vi "Convert ITX Experiment Folder.vi"(8 "error in (no error)":errorcluster, 11 "Folder Path":path) -> (0 "error out":errorcluster)   [LabVIEW 2016, in "Conversion.lvclass"]
uses:
  Conversion.lvclass
  Conversion.lvclass/Conversion.ctl
  Data/Data.lvclass
panel:
  in  "OK":bool
  in  "Additional Notes?":string
  out "Elapsed Time (s)":dbl
  out "Numeric":i32
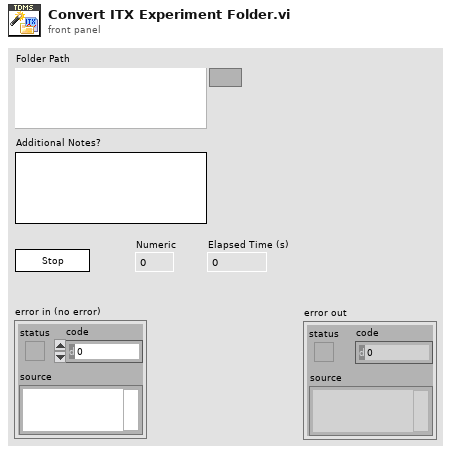
[diagram p1: front panel]
types:
  T1 = enum32{"Invalid", "Standard", "Closed", "Hidden", "Minimized", "Maximized"}
  T2 = enum32{"invalid app kind", "Development System", "Run Time System", "Student Edition", "Embedded LabVIEW", "Evaluation", "Custom"}
  T3 = cluster{"Core":cluster{"Current VI Reference":refnum<vi>, "Close Panel on Exit?":bool}, "Conversion.lvclass":refnum<class "Conversion.lvclass">, "Start Time":dbl, "End Time":dbl, "File Index":i32, "Number of Files":i32, "Log File Path":path}
  T4 = cluster{"Current VI Reference":refnum<vi>, "Close Panel on Exit?":bool}
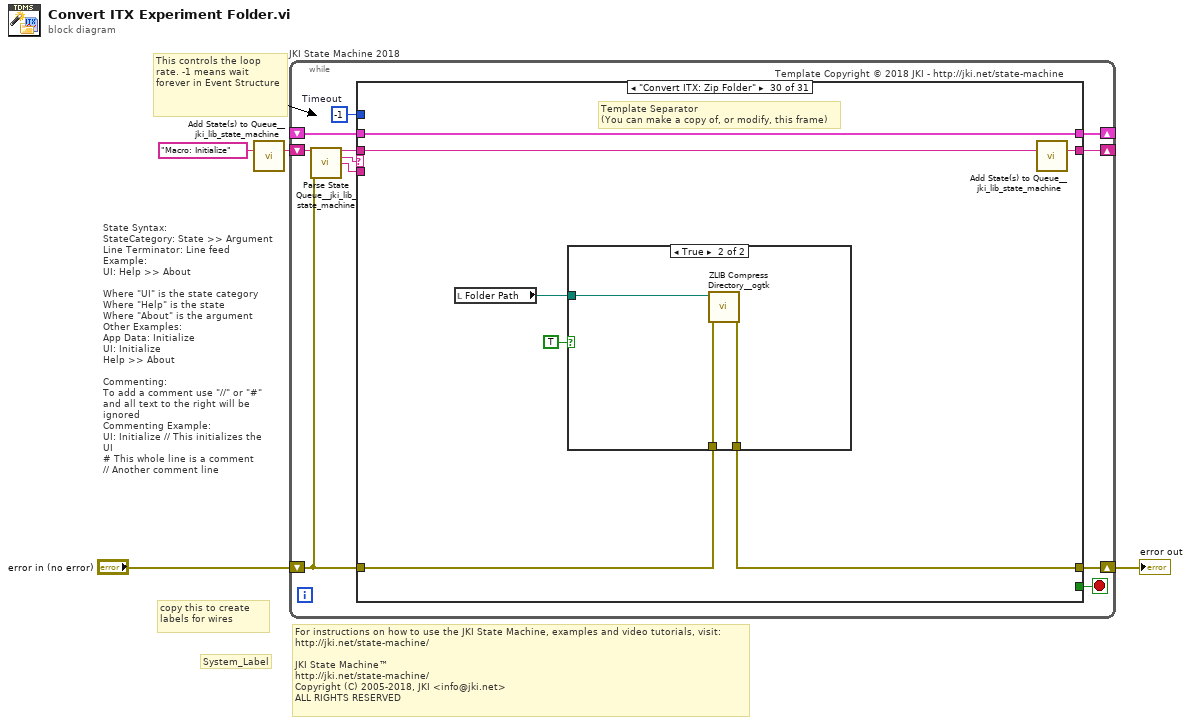
[diagram p0: block diagram]
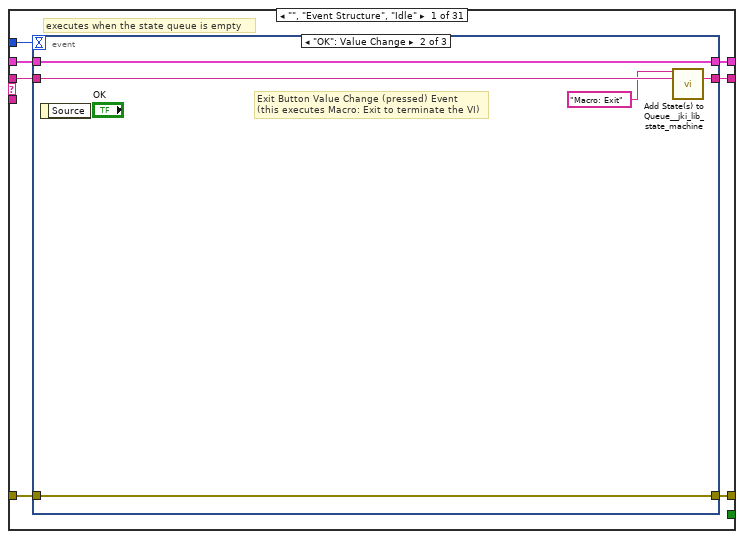
[diagram p2: hidden frame]
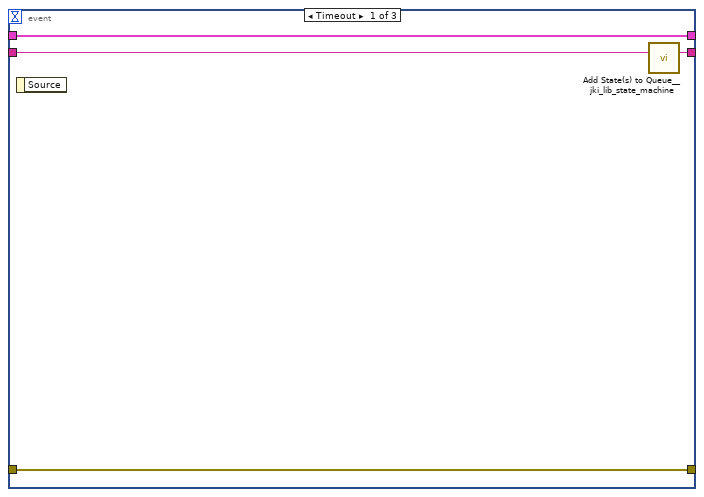
[diagram p3: hidden frame]
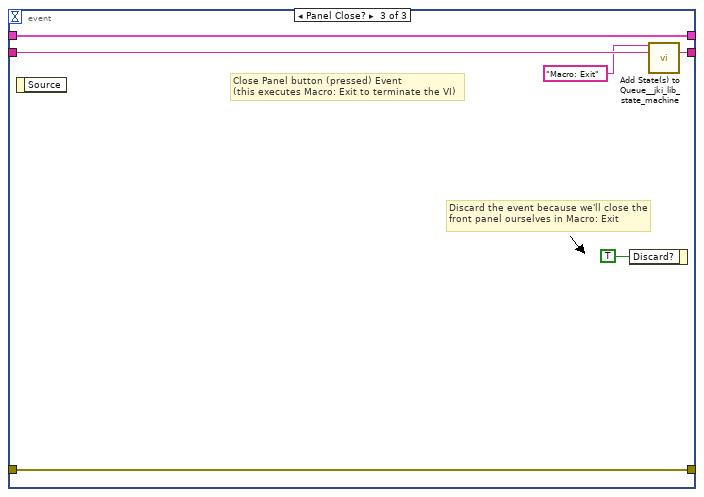
[diagram p4: hidden frame]
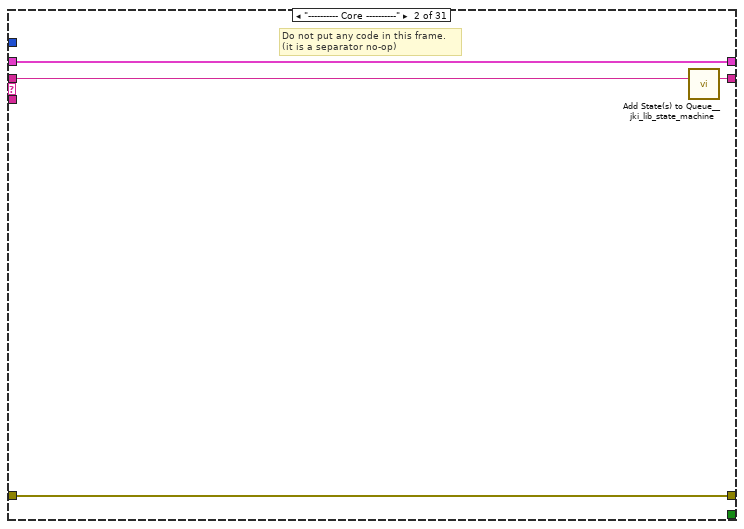
[diagram p5: hidden frame]
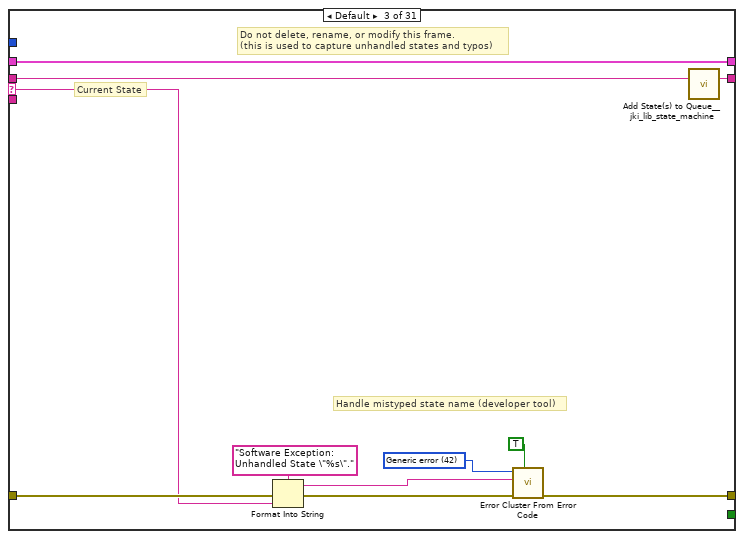
[diagram p6: hidden frame]
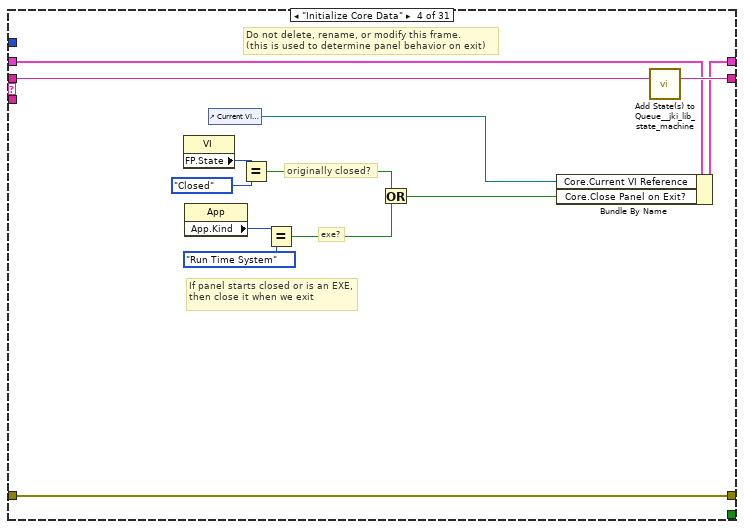
[diagram p7: hidden frame]
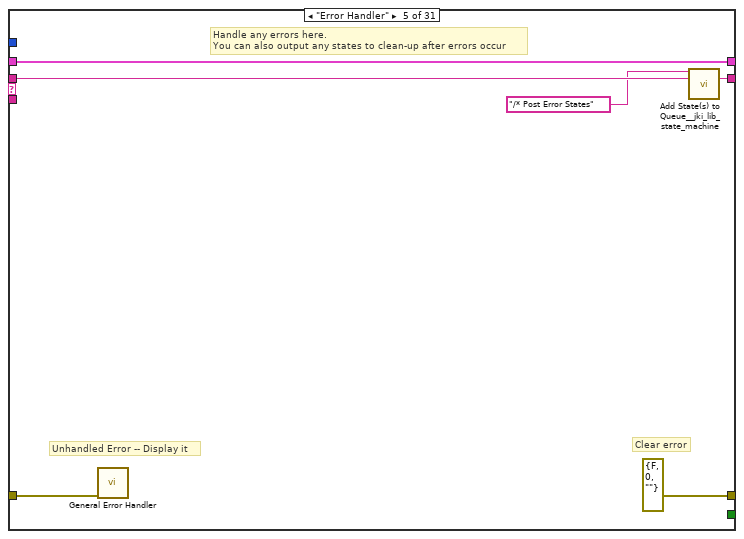
[diagram p8: hidden frame]
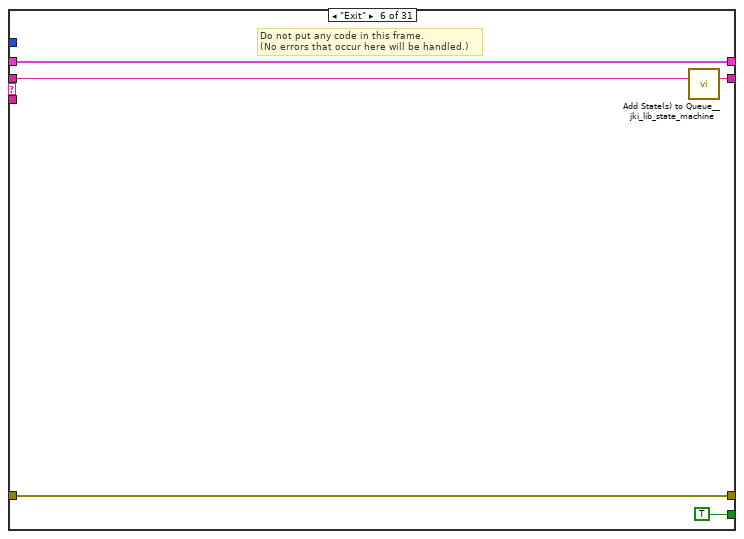
[diagram p9: hidden frame]
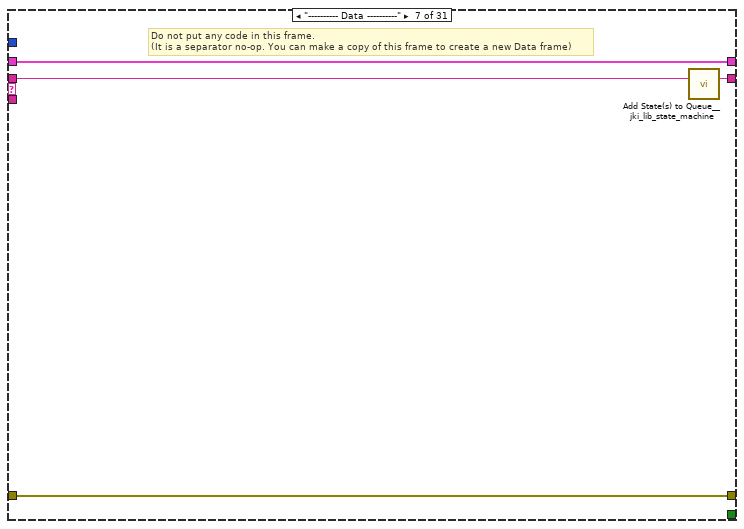
[diagram p10: hidden frame]
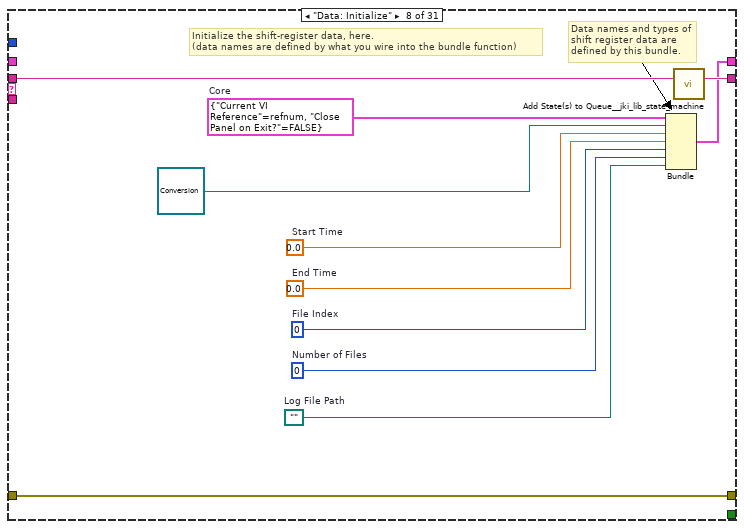
[diagram p11: hidden frame]
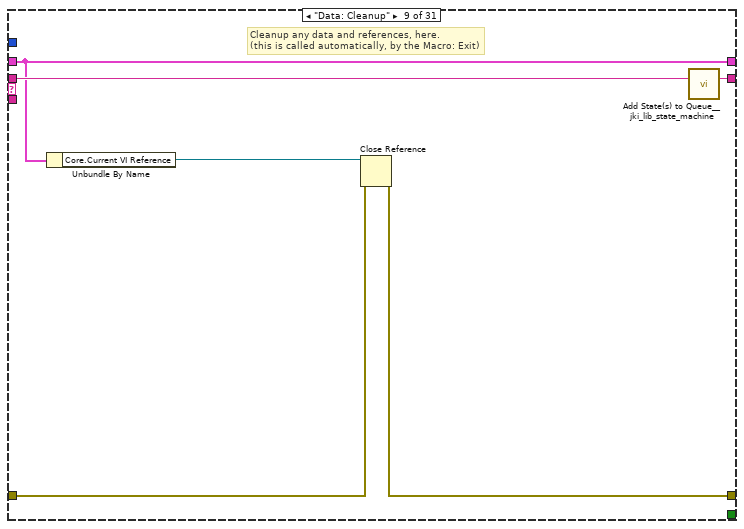
[diagram p12: hidden frame]
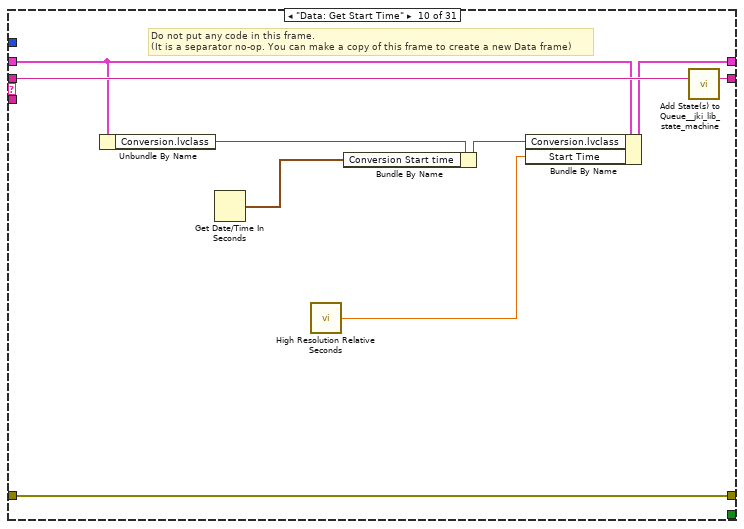
[diagram p13: hidden frame]
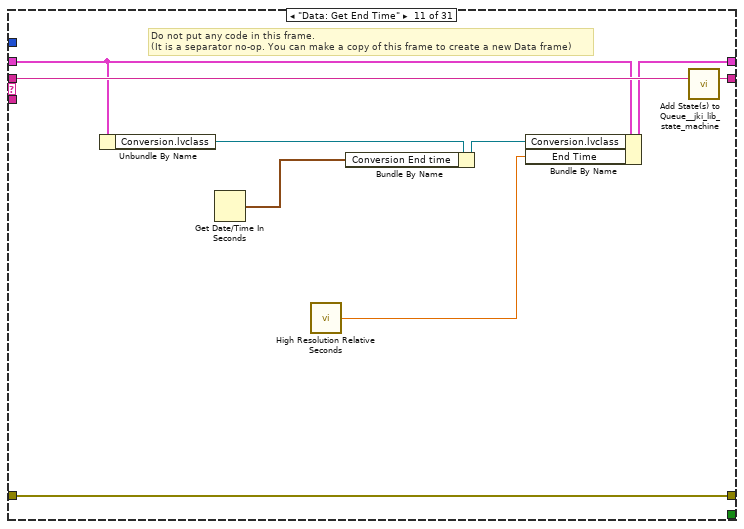
[diagram p14: hidden frame]
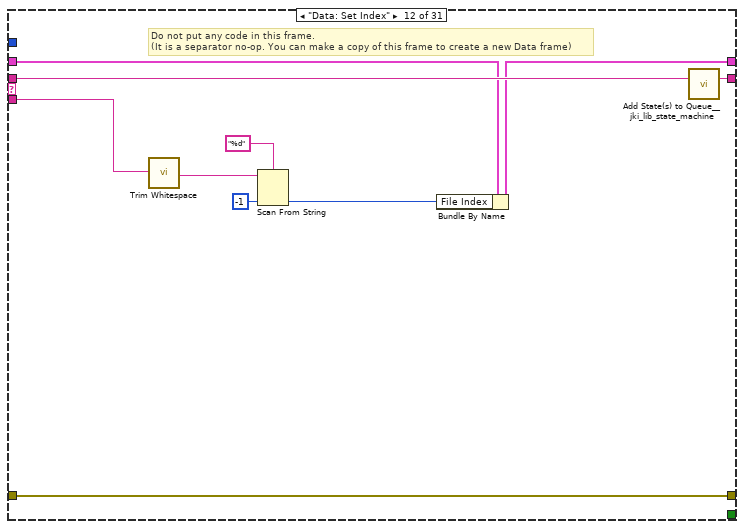
[diagram p15: hidden frame]
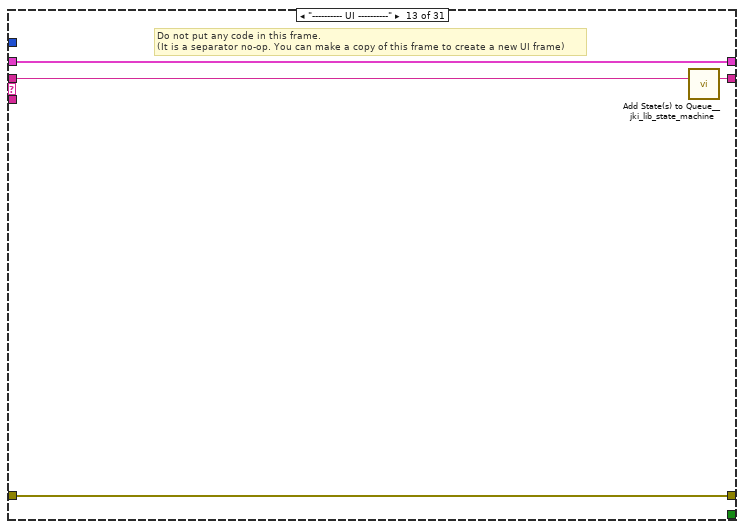
[diagram p16: hidden frame]
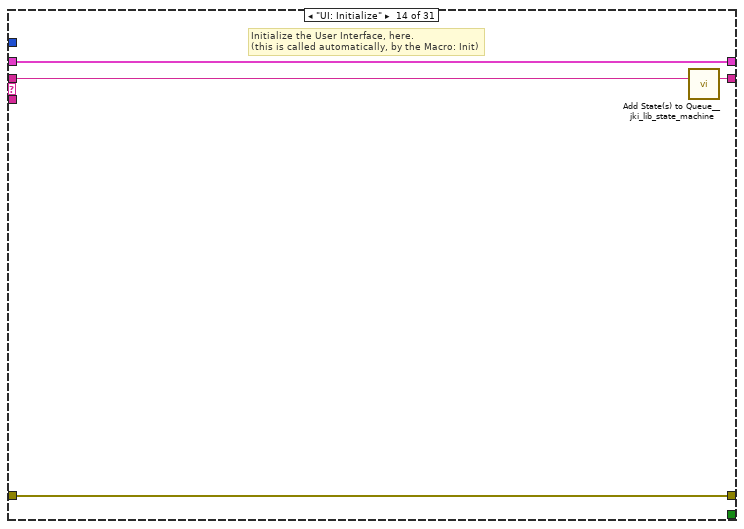
[diagram p17: hidden frame]
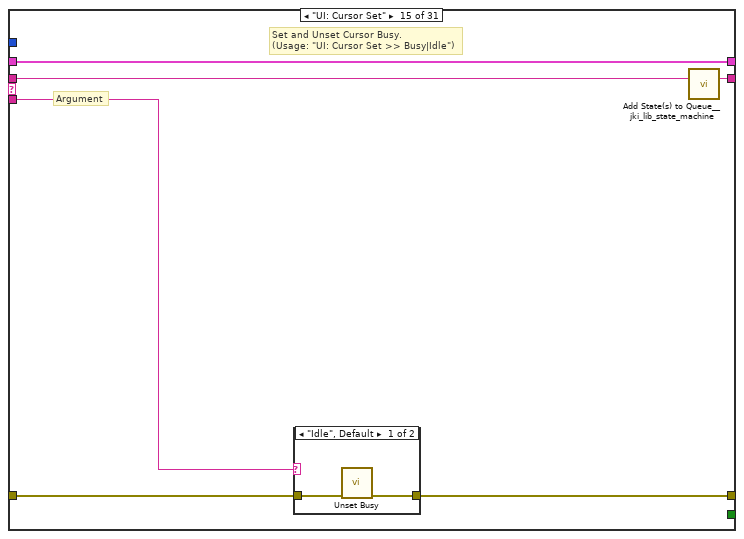
[diagram p18: hidden frame]
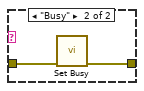
[diagram p19: hidden frame]
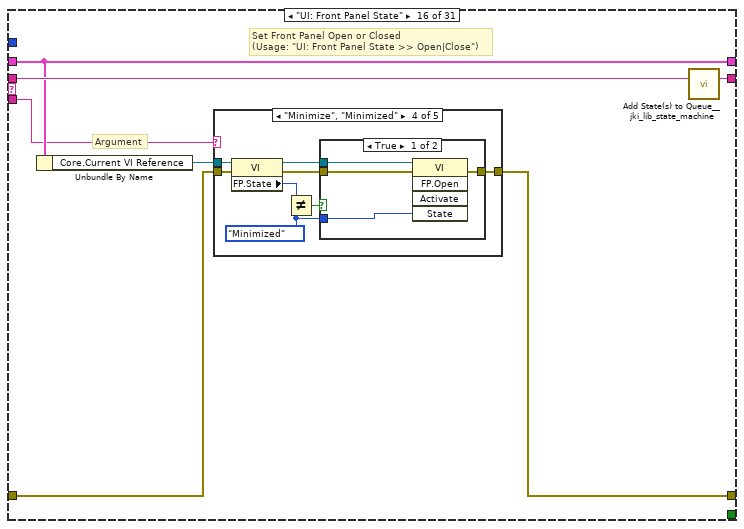
[diagram p20: hidden frame]
diagram:
  # "For instructions on how to use the JKI State Machine, examples and video tutorials, visit:\nhttp://jki.net/state-machine/\n\nJKI State Machine™\nhttp://jki.net/state-machine/\nCopyright (C) 2005-2018, JKI <info@jki.net>\nALL RIGHTS RESERVED"
  # "State Syntax:\nStateCategory: State >> Argument\nLine Terminator: Line feed\nExample:\nUI: Help >> About\n\nWhere \"UI\" is the state category\nWhere \"Help\" is the state\nWhere \"About\" is the argument\nOther Examples:\nApp Data: Initialize\nUI: Initialize\nHelp >> About\n\nCommenting:\nTo add a comment use \"//\" or \"#\" and all text to the right will be ignored\nCommenting Example:\nUI: Initialize // This initializes the UI\n# This whole line is a comment\n// Another comment line"
  # "copy this to create labels for wires"
  # "This controls the loop rate. -1 means wait forever in Event Structure"
  # "System_Label"
  n1 = call <vilib>:"Add State(s) to Queue__jki_lib_state_machine.vi"("State(s) in (\"\")"="Macro: Initialize") -> ("States Out"=w4:string)  [unwired: 14 in]
  n2 = while "JKI State Machine 2018" {
    shift-right: [w8] -> _
    shift-left: _ -> [w7]
    shift-right: [w11] -> w1
    shift-left: "error in (no error)" -> [w5]
    shift-right: [w10] -> _
    shift-left: w4 -> [w12]
    stop <- w9 stop-if-true
    w6 = -1  # Timeout
    # "Template Copyright © 2018 JKI - http://jki.net/state-machine"
    n3 = call <vilib>:"Parse State Queue__jki_lib_state_machine.vi"("State Queue"=w12, "Error In (no error)"=w5) -> ("Remaining States"=w14:string, "Current State"=w15:string, "Arguments"=w13:string)  [unwired: 11 in]
    n4 = case shown="\"Convert ITX: Zip Folder\"" w15 {
      selector: w15 -> [_ _ w42 _ _ _ _ _ _ _ _ _ _ _ _ _ _ _ _ _ _ _ _ _ _ _ _ _ _ _ _]
      tunnel: w14 -> [w22 w41 w46 w65 w71 w76 w80 w91 w97 w106 w115 w125 w129 w133 w139 w150 w222 w227 w231 w236 w241 w257 w262 w272 w276 w287 w298 w305 w315 w322 w341]
      tunnel: w13 -> [_ _ _ _ _ _ _ _ _ _ _ w116 _ _ w134 w144 _ _ _ _ _ _ _ _ _ _ _ _ _ _ _]
      tunnel: w7 -> [w20 w38 w44 w58 w68 w74 w77 _ w92 w103 w112 w121 w126 w131 w137 w146 w219 w224 w228 w233 w238 w245 w259 w269 w273 w283 w291 w301 w309 w320 w337]
      tunnel: [w19 w39 w48 w62 errorcluster {"status"=FALSE, "code"=0, "source"=""} ("error out") w73 w78 w88 w93 w104 w113 w123 w127 w130 w135 w147 w220 w225 w229 w234 w239 w255 w260 w270 w274 w279 w296 w299 w311 w318 w331] -> w11
      tunnel: w5 -> [w18 w39 w47 w62 w67 w73 w78 w88 w94 w104 w113 w123 w127 w130 w136 w148 w220 w225 w229 w234 w239 w255 w260 w270 w274 w280 w294 w300 w312 w319 w332]
      tunnel: [w21 w40 w45 w64 w70 w75 w79 w90 w96 w105 w114 w124 w128 w132 w138 w149 w221 w226 w230 w235 w240 w256 w261 w271 w275 w286 w297 w304 w314 w321 w340] -> w10
      tunnel: [_ _ _ _ _ TRUE _ _ _ _ _ _ _ _ _ _ _ _ _ _ _ _ _ _ _ _ _ _ _ _ _] -> w9
      tunnel: [w17 w38 w44 w63 w68 w74 w77 w89 w92 w102 w111 w122 w126 w131 w137 w146 w219 w224 w228 w233 w238 w245 w259 w269 w273 w282 w290 w301 w308 w320 w337] -> w8
      tunnel: w6 -> [w16 _ _ _ _ _ _ _ _ _ _ _ _ _ _ _ _ _ _ _ _ _ _ _ _ _ _ _ _ _ _]
      frame "", "Event Structure", "Idle" {
        # "executes when the state queue is empty"
        n5 = event shown="[1] \"OK\": Value Change" {
          selector: _ -> [_ _ _]
          dyn-events: _ -> [_ _ _]
          timeout: w16 -> [_ _ _]
          tunnel: w22 -> [w26 w31 w37]
          tunnel: [w25 w30 w36] -> w21
          tunnel: w20 -> [w24 w28 w34]
          tunnel: [w23 w29 w35] -> w19
          tunnel: w18 -> [w23 w29 w35]
          tunnel: [w24 w28 w34] -> w17
          event Timeout {
            n6 = event-data() -> ()  [unwired: 1 in, 1 out]
            n7 = call <vilib>:"Add State(s) to Queue__jki_lib_state_machine.vi"("State(s) in (\"\")"=w26) -> ("States Out"=w25:string)  [unwired: 14 in]
          }
          event "OK": Value Change {
            # "Exit Button Value Change (pressed) Event\n(this executes Macro: Exit to terminate the VI)"
            n8 = event-data() -> ()  [unwired: 1 in, 1 out]
            n9 = call <vilib>:"Add State(s) to Queue__jki_lib_state_machine.vi"("State(s) in Front (\"\")"="Macro: Exit", "State(s) in (\"\")"=w31) -> ("States Out"=w30:string)  [unwired: 13 in]
          }
          event Panel Close? {
            # "Discard the event because we'll close the front panel ourselves in Macro: Exit"
            # "Close Panel button (pressed) Event\n(this executes Macro: Exit to terminate the VI)"
            n10 = event-data() -> ()  [unwired: 1 in, 1 out]
            n11 = event-data("Discard?"=TRUE) -> ()  [unwired: 1 in, 1 out]
            n12 = call <vilib>:"Add State(s) to Queue__jki_lib_state_machine.vi"("State(s) in Front (\"\")"="Macro: Exit", "State(s) in (\"\")"=w37) -> ("States Out"=w36:string)  [unwired: 13 in]
          }
        }
      }
      frame "---------- Core ----------" {
        # "Do not put any code in this frame.\n(it is a separator no-op)"
        n13 = call <vilib>:"Add State(s) to Queue__jki_lib_state_machine.vi"("State(s) in (\"\")"=w41) -> ("States Out"=w40:string)  [unwired: 14 in]
      }
      frame Default {
        w51 = 42 items=["No error", "Argument error", "Memory is full", "Out of zone", "End of file", "File already open", "Generic file I/O error", "File not found", "File permission error", "Disk is full", "Duplicate path", "Too many files open", "System feature not enabled", "Resource file not found", "Cannot add resource", "Resource not found", "Image not found", "Image memory error", "Pen does not exist", "Config type invalid", "Config token not found", "Config parse error", "Config memory error", "Bad external code format", "Bad external code offset", "External code not present", "Null window", "Destroy window error", "Null menu", "Print aborted", "Bad print record", "Print driver error", "Windows error during printing", "Memory error during printing", "Print dialog error", "Generic print error", "Invalid device refnum", "Device not found", "Device parameter error", "Device unit error", "Cannot open device", "Device call aborted", "Generic error", "Cancelled by user", "Object ID too low", "Object ID too high", "Object not in heap", "Unknown heap", "Unknown object (invalid DefProc)", "Unknown object (DefProc not in table)", "Message out of range", "Invalid (null) method", "Unknown message", "Manager call not supported", "Bad address", "Network operation in progress", "Network operation timed out", "Connection is busy", "Network attribute not supported", "Network error", "Address in use", "System out of memory", "Connection aborted", "Connection refused", "Not connected", "Already connected", "Connection closed", "Initialization error (interapplication manager)", "Bad occurrence", "Wait on unbound occurrence handler", "Occurrence queue overflow", "Datalog type conflict", "Unused", "Unrecognized type (interapplication manager)", "Memory corrupt", "Failed to make temporary DLL", "Old CIN version", "Drag socket not found", "Failed to load drop-object", "Failed to register OLE object", "Failed to release OLE object", "Format specifier type mismatch", "Unknown format specifier", "Too few format specifiers", "Too many format specifiers", "Scan failed", "Newer CIN version", "Error converting to variant", "Runtime menu error", "Password tampered", "Variant attribute not found", "Incompatible variant data type", "Event data is not available", "Event Store is not present", "Occurrence is not found", "Event Queue is not created", "Event info is not available", "Refnum passed is NULL", "Error retrieving Class GUID", "Error retrieving CoClass GUID", "Error retrieving TypeLib GUID.", "Bad built application magic bytes.", "Specific driver is different from the specific driver associated with the Logical Name.", "There is no session opened to the class driver.", "Max Error", "MAX - Error with config objects", "MAX - Error loading configuration", "MAX - Group not supported"]
        # "Current State"
        # "Do not delete, rename, or modify this frame.\n(this is used to capture unhandled states and typos)"
        # "Handle mistyped state name (developer tool)"
        n14 = Format Into String(format string="Software Exception: Unhandled State \"%s\"." ("message"), error in=w47, w42) -> (resulting string=w50:string, error out=w49:errorcluster)  [unwired: 1 in]
        n15 = call <vilib>:"Error Cluster From Error Code.vi"("show call chain? (False)"=TRUE, "error in (no error)"=w49, "error message (\"\")"=w50, "error code (0)"=w51) -> ("error out"=w48:errorcluster)  [unwired: 5 in]
        n16 = call <vilib>:"Add State(s) to Queue__jki_lib_state_machine.vi"("State(s) in (\"\")"=w46) -> ("States Out"=w45:string)  [unwired: 14 in]
      }
      frame "Initialize Core Data" {
        # "Do not delete, rename, or modify this frame.\n(this is used to determine panel behavior on exit)"
        # "originally closed?"
        # "exe?"
        # "If panel starts closed or is an EXE, then close it when we exit"
        n17 = property class="VI"() -> ("FP.State"=w55:T1)  [unwired: 2 in, 2 out]
        n18 = property class="App"() -> ("App.Kind"=w61:T2)  [unwired: 2 in, 2 out]
        n19 = control-ref of="Current VI Reference"() -> (w56:refnum<vi>)
        n20 = Equal?(x=w55, y=T1."Closed" ("Front Panel Window:State")) -> (x = y?=w53:bool)
        n21 = Equal?(x=w61, y=T2."Run Time System" ("Application:Kind")) -> (x = y?=w59:bool)
        n22 = Or(x=w53, y=w59) -> (x .or. y?=w57:bool)
        n23 = Bundle By Name(cluster=w58, "Core.Current VI Reference"=w56, "Core.Close Panel on Exit?"=w57) -> (w63:T3)
        n24 = call <vilib>:"Add State(s) to Queue__jki_lib_state_machine.vi"("State(s) in (\"\")"=w65) -> ("States Out"=w64:string)  [unwired: 14 in]
      }
      frame "Error Handler" {
        # "Unhandled Error -- Display it"
        # "Handle any errors here.\nYou can also output any states to clean-up after errors occur"
        # "Clear error"
        n25 = call <vilib>:"General Error Handler.vi"("error in (no error)"=w67) -> ()  [unwired: 10 in, 5 out]
        n26 = call <vilib>:"Add State(s) to Queue__jki_lib_state_machine.vi"("State(s) in Front (\"\")"="/* Post Error States", "State(s) in (\"\")"=w71) -> ("States Out"=w70:string)  [unwired: 13 in]
      }
      frame "Exit" {
        # "Do not put any code in this frame.\n(No errors that occur here will be handled.)"
        n27 = call <vilib>:"Add State(s) to Queue__jki_lib_state_machine.vi"("State(s) in (\"\")"=w76) -> ("States Out"=w75:string)  [unwired: 14 in]
      }
      frame "---------- Data ----------" {
        # "Do not put any code in this frame.\n(It is a separator no-op. You can make a copy of this frame to create a new Data frame)"
        n28 = call <vilib>:"Add State(s) to Queue__jki_lib_state_machine.vi"("State(s) in (\"\")"=w80) -> ("States Out"=w79:string)  [unwired: 14 in]
      }
      frame "Data: Initialize" {
        w81 = path ""  # Log File Path
        w82 = 0  # Number of Files
        w83 = 0  # File Index
        w84 = 0.0  # End Time
        w85 = 0.0  # Start Time
        w87 = T4 {"Current VI Reference"=refnum, "Close Panel on Exit?"=FALSE}  # Core
        # "Data names and types of shift register data are defined by this bundle."
        # "Initialize the shift-register data, here.\n(data names are defined by what you wire into the bundle function)"
        n29 = Bundle("Core"=w87, "Conversion.lvclass"=refnum<class "Conversion.lvclass"> refnum, "Start Time"=w85, "End Time"=w84, "File Index"=w83, "Number of Files"=w82, "Log File Path"=w81) -> (w89:T3)  [unwired: 1 in]
        n30 = call <vilib>:"Add State(s) to Queue__jki_lib_state_machine.vi"("State(s) in (\"\")"=w91) -> ("States Out"=w90:string)  [unwired: 14 in]
      }
      frame "Data: Cleanup" {
        # "Cleanup any data and references, here.\n(this is called automatically, by the Macro: Exit)"
        n31 = Unbundle By Name(w92) -> ("Core.Current VI Reference"=w95:refnum<vi>)
        n32 = Close Reference(reference=w95, error in (no error)=w94) -> (error out=w93:errorcluster)
        n33 = call <vilib>:"Add State(s) to Queue__jki_lib_state_machine.vi"("State(s) in (\"\")"=w97) -> ("States Out"=w96:string)  [unwired: 14 in]
      }
      frame "Data: Get Start Time" {
        # "Do not put any code in this frame.\n(It is a separator no-op. You can make a copy of this frame to create a new Data frame)"
        n34 = Unbundle By Name(w103) -> ("Conversion.lvclass"=w100:refnum<class "Conversion.lvclass">)
        n35 = Get Date/Time In Seconds() -> (seconds since 1Jan1904=w101:timestamp)
        n36 = call <vilib>:"High Resolution Relative Seconds.vi"() -> ("relative seconds"=w98:dbl)
        n37 = Bundle By Name(cluster=w100, "Conversion Start time"=w101) -> (w99:refnum<class "Conversion.lvclass">)
        n38 = Bundle By Name(cluster=w103, "Conversion.lvclass"=w99, "Start Time"=w98) -> (w102:T3)
        n39 = call <vilib>:"Add State(s) to Queue__jki_lib_state_machine.vi"("State(s) in (\"\")"=w106) -> ("States Out"=w105:string)  [unwired: 14 in]
      }
      frame "Data: Get End Time" {
        # "Do not put any code in this frame.\n(It is a separator no-op. You can make a copy of this frame to create a new Data frame)"
        n40 = Unbundle By Name(w112) -> ("Conversion.lvclass"=w109:refnum<class "Conversion.lvclass">)
        n41 = Get Date/Time In Seconds() -> (seconds since 1Jan1904=w110:timestamp)
        n42 = call <vilib>:"High Resolution Relative Seconds.vi"() -> ("relative seconds"=w107:dbl)
        n43 = Bundle By Name(cluster=w109, "Conversion End time"=w110) -> (w108:refnum<class "Conversion.lvclass">)
        n44 = Bundle By Name(cluster=w112, "Conversion.lvclass"=w108, "End Time"=w107) -> (w111:T3)
        n45 = call <vilib>:"Add State(s) to Queue__jki_lib_state_machine.vi"("State(s) in (\"\")"=w115) -> ("States Out"=w114:string)  [unwired: 14 in]
      }
      frame "Data: Set Index" {
        # "Do not put any code in this frame.\n(It is a separator no-op. You can make a copy of this frame to create a new Data frame)"
        n46 = call <vilib>:"Trim Whitespace.vi"("string"=w116) -> ("trimmed string"=w120:string)  [unwired: 1 in]
        n47 = Scan From String(format string="%d", input string=w120, default 1=-1 ("default value 1")) -> (output 1=w117:i32)  [unwired: 2 in, 3 out]
        n48 = Bundle By Name(cluster=w121, "File Index"=w117) -> (w122:T3)
        n49 = call <vilib>:"Add State(s) to Queue__jki_lib_state_machine.vi"("State(s) in (\"\")"=w125) -> ("States Out"=w124:string)  [unwired: 14 in]
      }
      frame "---------- UI ----------" {
        # "Do not put any code in this frame.\n(It is a separator no-op. You can make a copy of this frame to create a new UI frame)"
        n50 = call <vilib>:"Add State(s) to Queue__jki_lib_state_machine.vi"("State(s) in (\"\")"=w129) -> ("States Out"=w128:string)  [unwired: 14 in]
      }
      frame "UI: Initialize" {
        # "Initialize the User Interface, here.\n(this is called automatically, by the Macro: Init)"
        n51 = call <vilib>:"Add State(s) to Queue__jki_lib_state_machine.vi"("State(s) in (\"\")"=w133) -> ("States Out"=w132:string)  [unwired: 14 in]
      }
      frame "UI: Cursor Set" {
        # "Argument"
        # "Set and Unset Cursor Busy.\n(Usage: \"UI: Cursor Set >> Busy|Idle\")"
        n52 = case shown="\"Idle\", Default" w134 {
          tunnel: w136 -> [w141 w143]
          tunnel: [w140 w142] -> w135
          frame "Idle", Default {
            n53 = call <vilib>:"Unset Busy.vi"("error in (no error)"=w141) -> ("error out"=w140:errorcluster)  [unwired: 10 in]
          }
          frame "Busy" {
            n54 = call <vilib>:"Set Busy.vi"("error in (no error)"=w143) -> ("error out"=w142:errorcluster)  [unwired: 9 in, 1 out]
          }
        }
        n55 = call <vilib>:"Add State(s) to Queue__jki_lib_state_machine.vi"("State(s) in (\"\")"=w139) -> ("States Out"=w138:string)  [unwired: 14 in]
      }
      frame "UI: Front Panel State" {
        # "Argument"
        # "Set Front Panel Open or Closed\n(Usage: \"UI: Front Panel State >> Open|Close\")"
        n56 = Unbundle By Name(w146) -> ("Core.Current VI Reference"=w145:refnum<vi>)
        n57 = case shown="\"Minimize\", \"Minimized\"" w144 {
          tunnel: w148 -> [w156 w171 w182 w195 w208]
          tunnel: [w158 w172 w184 w197 w210] -> w147
          tunnel: w145 -> [w157 w169 w183 w196 w209]
          frame "Open", "Standard", Default {
            w151 = T1."Standard" ("State")
            n58 = property class="VI"(reference=w157, error in=w156) -> (reference out=w154:refnum<vi>, error out=w155:errorcluster, "FP.State"=w153:T1)
            n59 = Not Equal?(x=w153, y=w151) -> (x != y?=w152:bool)
            n60 = case shown="True" w152 {
              tunnel: [w162 w164] -> w158
              tunnel: w155 -> [w161 w164]
              tunnel: w154 -> [w160 _]
              tunnel: w151 -> [w159 _]
              frame True {
                n61 = invoke class="VI" method="FP.Open"(reference=w160, error in=w161, "Activate"=TRUE, "State"=w159) -> (error out=w162:errorcluster)  [unwired: 1 in, 4 out]
              }
              frame False {
              }
            }
          }
          frame "Close", "Closed" {
            n62 = property class="VI"(reference=w169, error in=w171) -> (reference out=w168:refnum<vi>, error out=w170:errorcluster, "FP.State"=w166:T1)
            n63 = Not Equal?(x=w166, y=T1."Closed" ("Front Panel Window:State")) -> (x != y?=w165:bool)
            n64 = case shown="True" w165 {
              tunnel: [w173 w176] -> w172
              tunnel: w170 -> [w173 w175]
              tunnel: w168 -> [_ w174]
              frame False {
              }
              frame True {
                n65 = invoke class="VI" method="FP.Close"(reference=w174, error in=w175) -> (error out=w176:errorcluster)  [unwired: 1 in, 2 out]
              }
            }
          }
          frame "Hidden", "Hide" {
            w177 = T1."Hidden" ("State")
            n66 = property class="VI"(reference=w183, error in=w182) -> (reference out=w180:refnum<vi>, error out=w181:errorcluster, "FP.State"=w179:T1)
            n67 = Not Equal?(x=w179, y=w177) -> (x != y?=w178:bool)
            n68 = case shown="True" w178 {
              tunnel: [w188 w189] -> w184
              tunnel: w181 -> [w187 w189]
              tunnel: w180 -> [w186 _]
              tunnel: w177 -> [w185 _]
              frame True {
                n69 = invoke class="VI" method="FP.Open"(reference=w186, error in=w187, "State"=w185) -> (error out=w188:errorcluster)  [unwired: 2 in, 4 out]
              }
              frame False {
              }
            }
          }
          frame "Minimize", "Minimized" {
            w190 = T1."Minimized" ("State")
            n70 = property class="VI"(reference=w196, error in=w195) -> (reference out=w193:refnum<vi>, error out=w194:errorcluster, "FP.State"=w192:T1)
            n71 = Not Equal?(x=w192, y=w190) -> (x != y?=w191:bool)
            n72 = case shown="True" w191 {
              tunnel: [w201 w202] -> w197
              tunnel: w194 -> [w200 w202]
              tunnel: w193 -> [w199 _]
              tunnel: w190 -> [w198 _]
              frame True {
                n73 = invoke class="VI" method="FP.Open"(reference=w199, error in=w200, "State"=w198) -> (error out=w201:errorcluster)  [unwired: 2 in, 4 out]
              }
              frame False {
              }
            }
          }
          frame "Maximize", "Maximized" {
            w203 = T1."Maximized" ("State")
            n74 = property class="VI"(reference=w209, error in=w208) -> (reference out=w206:refnum<vi>, error out=w207:errorcluster, "FP.State"=w205:T1)
            n75 = Not Equal?(x=w205, y=w203) -> (x != y?=w204:bool)
            n76 = case shown="True" w204 {
              tunnel: [w214 w215] -> w210
              tunnel: w207 -> [w213 w215]
              tunnel: w206 -> [w212 _]
              tunnel: w203 -> [w211 _]
              frame True {
                n77 = invoke class="VI" method="FP.Open"(reference=w212, error in=w213, "State"=w211) -> (error out=w214:errorcluster)  [unwired: 2 in, 4 out]
              }
              frame False {
              }
            }
          }
        }
        n78 = call <vilib>:"Add State(s) to Queue__jki_lib_state_machine.vi"("State(s) in (\"\")"=w150) -> ("States Out"=w149:string)  [unwired: 14 in]
      }
      frame "UI: Update Elapsed Time" {
        # "Do not put any code in this frame.\n(It is a separator no-op. You can make a copy of this frame to create a new UI frame)"
        n79 = Unbundle By Name(w219) -> ("Start Time"=w218:dbl)
        n80 = call <vilib>:"High Resolution Relative Seconds.vi"() -> ("relative seconds"=w217:dbl)
        n81 = Subtract(x=w217, y=w218) -> (x-y=→"Elapsed Time (s)":dbl)
        n82 = call <vilib>:"Add State(s) to Queue__jki_lib_state_machine.vi"("State(s) in (\"\")"=w222) -> ("States Out"=w221:string)  [unwired: 14 in]
      }
      frame "UI: Update Index" {
        # "Do not put any code in this frame.\n(It is a separator no-op. You can make a copy of this frame to create a new UI frame)"
        n83 = Unbundle By Name(w224) -> ("File Index"=→"Numeric":i32)
        n84 = call <vilib>:"Add State(s) to Queue__jki_lib_state_machine.vi"("State(s) in (\"\")"=w227) -> ("States Out"=w226:string)  [unwired: 14 in]
      }
      frame "---------- Macro ----------" {
        # "Do not put any code in this frame.\n(It is a separator no-op. You can make a copy of this frame to create a new Macro frame)"
        n85 = call <vilib>:"Add State(s) to Queue__jki_lib_state_machine.vi"("State(s) in (\"\")"=w231) -> ("States Out"=w230:string)  [unwired: 14 in]
      }
      frame "Macro: Initialize" {
        w232 = "Data: Initialize\nInitialize Core Data\nUI: Initialize\nUI: Front Panel State >> Open\nMacro: Convert Initialize\nMacro: Convert"  # Data: Initialize Initialize Core Data UI: Initialize UI: Front Panel State >> Open Macro: Convert Initialize Macro: Convert
        # "Initialization Macro\n(This is called once, when the VI starts)"
        n86 = call <vilib>:"Add State(s) to Queue__jki_lib_state_machine.vi"("State(s) in Front (\"\")"=w232, "State(s) in (\"\")"=w236) -> ("States Out"=w235:string)  [unwired: 13 in]
      }
      frame "Macro: Convert Initialize" {
        # "Initialization Macro\n(This is called once, when the VI starts)"
        n87 = call <vilib>:"Add State(s) to Queue__jki_lib_state_machine.vi"("State(s) in Front (\"\")"="\nData: Set Index >> 0\nConvert ITX: Get Files\nData: Get Start Time\nUI: Update Index\nUI: Update Elapsed Time", "State(s) in (\"\")"=w241) -> ("States Out"=w240:string)  [unwired: 13 in]
      }
      frame "Macro: Convert" {
        # "Still Running?\n(OR are we done?)"
        # "next step"
        # "Initialization Macro\n(This is called once, when the VI starts)"
        n88 = Unbundle By Name(w245) -> ("File Index"=w249:i32, "Conversion.lvclass"=w244:refnum<class "Conversion.lvclass">)
        n89 = Unbundle By Name(w244) -> ("Original"=w243:path[])
        n90 = Increment(x=w249) -> (x+1=w246:i32)
        n91 = Array Size(array=w243) -> (size(s)=w253:i32)
        n92 = Decrement(x=w253) -> (x-1=w254:i32)
        n93 = In Range and Coerce(upper limit=w254, x=w246, lower limit=0) -> (In Range?=w251:bool)  [unwired: 1 out]
        n94 = Format Into String(format string="Data: Set Index >> %d\nUI: Update Index\nConvert ITX: ITX to TDMS\nUI: Update Elapsed Time\n\nMacro: Convert", w246) -> (resulting string=w248:string)  [unwired: 2 in, 1 out]
        n95 = Select(t=w248, s=w251, f="Macro: Convert Cleanup ") -> (s? t:f=w242:string)
        n96 = call <vilib>:"Add State(s) to Queue__jki_lib_state_machine.vi"("State(s) in Front (\"\")"=w242, "State(s) in (\"\")"=w257) -> ("States Out"=w256:string)  [unwired: 13 in]
      }
      frame "Macro: Convert Cleanup" {
        # "Initialization Macro\n(This is called once, when the VI starts)"
        n97 = call <vilib>:"Add State(s) to Queue__jki_lib_state_machine.vi"("State(s) in Front (\"\")"="Convert ITX: Close File\nData: Get End Time\nConvert ITX: Write Log File\nConvert ITX: Display Error\nMacro: Exit", "State(s) in (\"\")"=w262) -> ("States Out"=w261:string)  [unwired: 13 in]
      }
      frame "Macro: Exit" {
        # "Exit Macro\n(This is called once, when the VI exits)"
        n98 = Unbundle By Name(w269) -> ("Core.Close Panel on Exit?"=w268:bool)
        n99 = Select(t="UI: Front Panel State >> Close", s=w268, f="") -> (s? t:f=w265:string)
        n100 = call <vilib>:"Add State(s) to Queue__jki_lib_state_machine.vi"("State(s) in (\"\")"=w265, "State(s) at Back (\"\")"="Data: Cleanup\nExit") -> ("States Out"=w263:string)  [unwired: 13 in]
        n101 = call <vilib>:"Add State(s) to Queue__jki_lib_state_machine.vi"("State(s) in Front (\"\")"=w263, "State(s) in (\"\")"=w272) -> ("States Out"=w271:string)  [unwired: 13 in]
      }
      frame "---------- Convert ITX ----------" {
        # "Template Separator\n(You can make a copy of, or modify, this frame)"
        n102 = call <vilib>:"Add State(s) to Queue__jki_lib_state_machine.vi"("State(s) in (\"\")"=w276) -> ("States Out"=w275:string)  [unwired: 14 in]
      }
      frame "Convert ITX: Get Files" {
        # "Your code here.\n(You can make a copy of, or modify, this frame)"
        n103 = Unbundle By Name(w283) -> ("Conversion.lvclass"=w284:refnum<class "Conversion.lvclass">)
        n104 = call <vilib>:"Recursive File List.vi"("pattern"="*.itx", "error in (no error)"=w280, "Folder Path"="Folder Path") -> ("error out"=w279:errorcluster, "All Files in Dir"=w281:path[])  [unwired: 4 in, 3 out]
        n105 = Bundle By Name(cluster=w284, "Original"=w281) -> (w277:refnum<class "Conversion.lvclass">)
        n106 = Bundle By Name(cluster=w283, "Conversion.lvclass"=w277) -> (w282:T3)
        n107 = call <vilib>:"Add State(s) to Queue__jki_lib_state_machine.vi"("State(s) in (\"\")"=w287) -> ("States Out"=w286:string)  [unwired: 14 in]
      }
      frame "Convert ITX: ITX to TDMS" {
        # "Template Separator\n(You can make a copy of, or modify, this frame)"
        n108 = Unbundle By Name(w291) -> ("Conversion.lvclass"=w289:refnum<class "Conversion.lvclass">, "File Index"=w288:i32)
        n109 = Unbundle By Name(w289) -> ("Original"=w295:path[])
        n110 = Index Array(array=w295, index=w288) -> (element=w293:path)
        n111 = call "ITX to TDMS.vi"("error in (no error)"=w294, "Path"=w293, "Conversion.lvclass"=w289) -> ("error out"=w296:errorcluster, "Conversion.lvclass out"=w292:refnum<class "Conversion.lvclass">)  [unwired: 6 in, 1 out]
        n112 = Bundle By Name(cluster=w291, "Conversion.lvclass"=w292) -> (w290:T3)
        n113 = call <vilib>:"Add State(s) to Queue__jki_lib_state_machine.vi"("State(s) in (\"\")"=w298) -> ("States Out"=w297:string)  [unwired: 14 in]
      }
      frame "Convert ITX: Close File" {
        # "Template Separator\n(You can make a copy of, or modify, this frame)"
        n114 = Unbundle By Name(w301) -> ("Conversion.lvclass"=w303:refnum<class "Conversion.lvclass">)
        n115 = Unbundle By Name(w303) -> ("Data.lvclass"=w302:refnum<class "Data.lvclass">)
        n116 = call-dynamic "Close.vi"("error in (no error)"=w300, "Data in"=w302) -> ("error out"=w299:errorcluster)  [unwired: 8 in, 1 out]
        n117 = call <vilib>:"Add State(s) to Queue__jki_lib_state_machine.vi"("State(s) in (\"\")"=w305) -> ("States Out"=w304:string)  [unwired: 14 in]
      }
      frame "Convert ITX: Write Log File" {
        # "Your code here.\n(You can make a copy of, or modify, this frame)"
        n118 = Unbundle By Name(w309) -> ("Conversion.lvclass"=w310:refnum<class "Conversion.lvclass">)
        n119 = call "Write Conversion Log File.vi"("error in (no error)"=w312, "Additional Notes?"="Additional Notes?", "Conversion.lvclass"=w310) -> ("error out"=w311:errorcluster, "Log File Path"=w306:path, "Conversion.lvclass out"=w307:refnum<class "Conversion.lvclass">)  [unwired: 6 in]
        n120 = Bundle By Name(cluster=w309, "Conversion.lvclass"=w307, "Log File Path"=w306) -> (w308:T3)
        n121 = call <vilib>:"Add State(s) to Queue__jki_lib_state_machine.vi"("State(s) in (\"\")"=w315) -> ("States Out"=w314:string)  [unwired: 14 in]
      }
      frame "Convert ITX: Zip Folder" {
        # "Template Separator\n(You can make a copy of, or modify, this frame)"
        n122 = local read "Folder Path"() -> (w316:path)
        n123 = case shown="True" TRUE {
          tunnel: w319 -> [w327 w330]
          tunnel: [w326 w329] -> w318
          tunnel: w316 -> [w323 w328]
          frame False {
            n124 = Strip Path(path=w323) -> (stripped path=w324:path)  [unwired: 1 out]
            n125 = call <vilib>:"System Exec.vi"("error in (no error)"=w327, "working directory"=w324, "command line"="7z.exe something") -> ("error out"=w326:errorcluster)  [unwired: 5 in, 3 out]
          }
          frame True {
            n126 = call <userlib>:"ZLIB Compress Directory__ogtk.vi"("error in (no error)"=w330, "root directory (file dialog)"=w328) -> ("error out"=w329:errorcluster)  [unwired: 7 in, 2 out]
          }
        }
        n127 = call <vilib>:"Add State(s) to Queue__jki_lib_state_machine.vi"("State(s) in (\"\")"=w322) -> ("States Out"=w321:string)  [unwired: 14 in]
      }
      frame "Convert ITX: Display Error" {
        # "dialog is shown if errors detected"
        # "Template Separator\n(You can make a copy of, or modify, this frame)"
        n128 = Unbundle By Name(w337) -> ("Conversion.lvclass"=w336:refnum<class "Conversion.lvclass">, "Log File Path"=w333:path)
        n129 = Unbundle By Name(w336) -> ("Failed Conversions"=w335:path[])
        n130 = Array Size(array=w335) -> (size(s)=w334:i32)
        n131 = Format Into String(format string="There was an issue with the file conversoin\nCheck the log file for details:\n%s", error in=w332, w333) -> (resulting string=w338:string, error out=w331:errorcluster)  [unwired: 1 in]
        n132 = case shown="0" w334 {
          tunnel: w338 -> [_ w342]
          frame 0 {
          }
          frame Default {
            n133 = One Button Dialog(message=w342) -> ()  [unwired: 1 in, 1 out]
          }
        }
        n134 = call <vilib>:"Add State(s) to Queue__jki_lib_state_machine.vi"("State(s) in (\"\")"=w341) -> ("States Out"=w340:string)  [unwired: 14 in]
      }
    }
  }
  "error out" <- w1
